vi "temperaturePanelView.vi"() -> ()   [LabVIEW 2014]
uses:
  <vilib>/LabVIEW Interface for Arduino/Type Defs/Board Type.ctl
  <vilib>/LabVIEW Interface for Arduino/Type Defs/Connection Type.ctl
  <vilib>/LabVIEW Interface for Arduino/Type Defs/Pin Mode.ctl
  <vilib>/LabVIEW Interface for Arduino/LabVIEW Interface for Arduino.lvlib
  Arduino/libraries/LIFA-DHT/DHT11.lvlib
panel:
  out "Estado del Ventilador2":bool
  out "Estado del Ventilador1":bool
  in  "Tipos de Velocidad Motor2":i8(knob) scale=0.0..3.0
  in  "Motor 2 PIN":dbl
  in  "Tipos de Velocidad Motor1":i8(knob) scale=0.0..3.0
  in  "Temperatura Considerada calor":i8
  in  "Motor 1 PIN":dbl
  out "Registro de temperatura":u8(graph)
  in  "DHT11 PIN":fxp<+,4,4>
  out "TF label":dbl
  out "Temperatura F":dbl(slide) scale=0.0..180.0
  out "TC label":dbl
  out "Temperatura C°":dbl(slide) scale=0.0..100.0
  in  "Delay":fxp<+,16,16>
  in  "stop":bool
  in  "VISA resource":refnum<visa-resource-name>
  # "Ventilador Inteligente"
  # "Arduino"
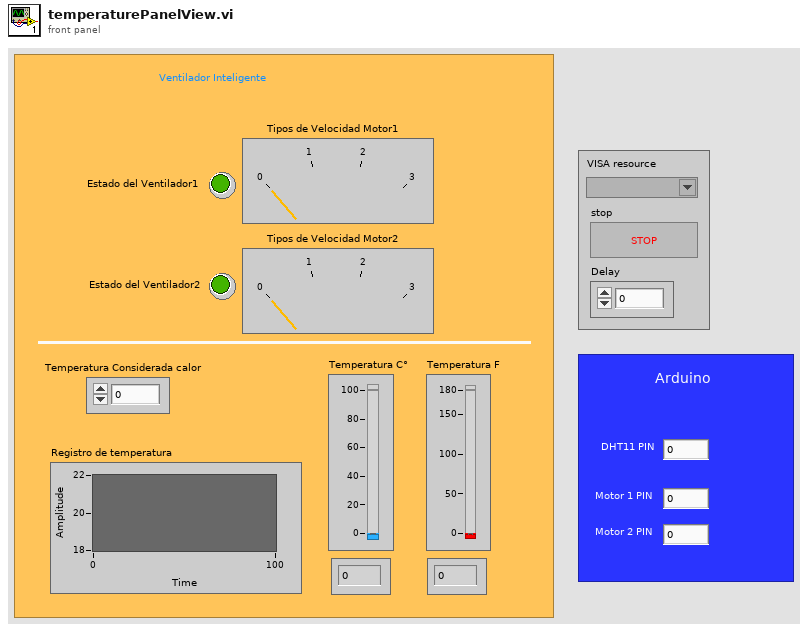
[diagram p1: front panel]
types:
  T1 = typedef "LabVIEW Interface for Arduino.lvlib/Pin Mode.ctl" = enum8{"Input", "Output"}
  T2 = typedef "LabVIEW Interface for Arduino.lvlib/Connection Type.ctl" = enum8{"USB / Serial", "XBEE", "BlueSmirf (Bluetooth)"}
  T3 = typedef "LabVIEW Interface for Arduino.lvlib/Board Type.ctl" = enum16{"Uno", "Dimuelanove w/Atmega 328", "Mega 2560"}
  T4 = typedef "LabVIEW Interface for Arduino.lvlib/Arduino Resource.ctl" = cluster{"VISA resource":refnum<visa-resource-name>, "Board Type":T3, "Connection Type":enum8{"USB / Serial"}, "Bytes Per Packet (15)":u8}
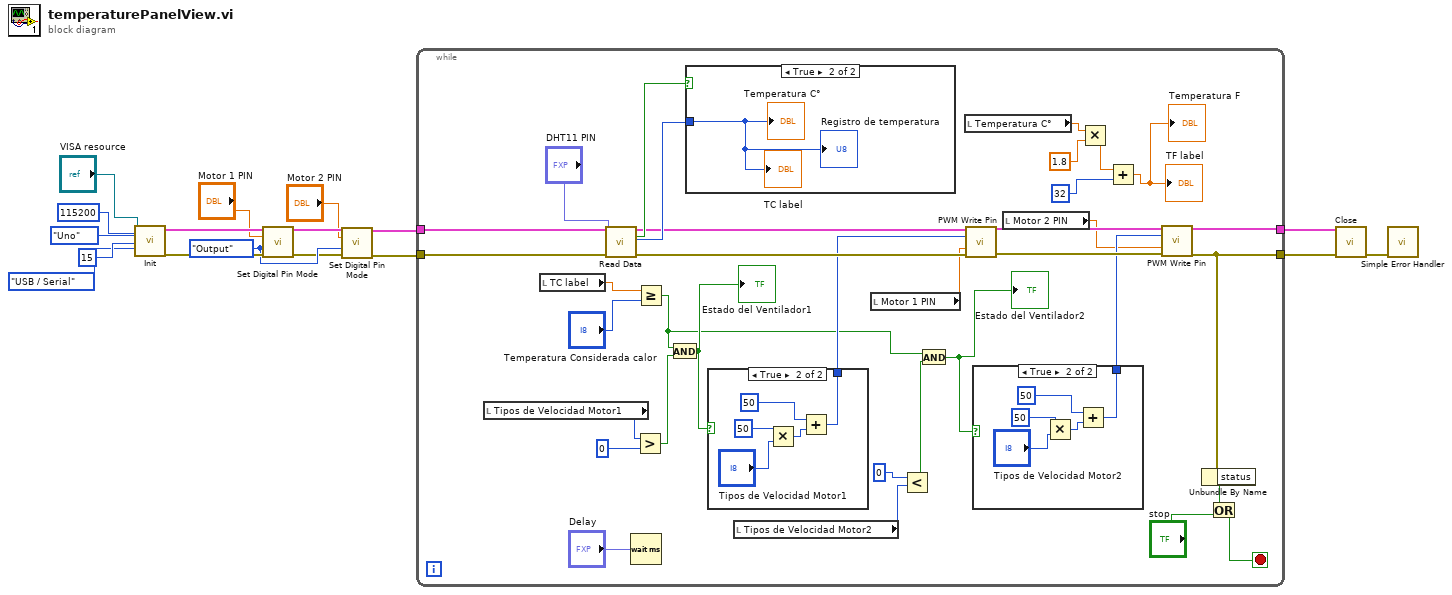
[diagram p0: block diagram]
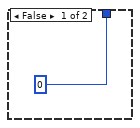
[diagram p2: hidden frame]
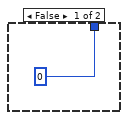
[diagram p3: hidden frame]
diagram:
  w4 = Pin_Mode."Output" ("Pin Mode (Input)")
  n1 = call <vilib>:"Init.vi"("VISA resource"="VISA resource", "Baud Rate (115200)"=u32 115200, "Board Type (Uno)"=Board_Type."Uno", "Bytes Per Packet (15)"=u32 15, "Connection Type (USB/Serial)"=Connection_Type."USB / Serial") -> ("Arduino Resource"=w9:T4, "error out"=w8:errorcluster)  [unwired: 13 in]
  n2 = call <vilib>:"Set Digital Pin Mode.vi"("Arduino Resource"=w9, "Digital I/O Pin"="Motor 1 PIN", "Pin Mode (Input)"=w4, "error in"=w8) -> ("Arduino Resource"=w6:T4, "error out"=w3:errorcluster)  [unwired: 10 in]
  n3 = call <vilib>:"Set Digital Pin Mode.vi"("Arduino Resource"=w6, "Digital I/O Pin"="Motor 2 PIN", "Pin Mode (Input)"=w4, "error in"=w3) -> ("Arduino Resource"=w5:T4, "error out"=w2:errorcluster)  [unwired: 10 in]
  n4 = while {
    tunnel: [w29] -> w12
    tunnel: [w28] -> w11
    tunnel: w5 -> [w48]
    tunnel: w2 -> [w47]
    stop <- w50 stop-if-true
    n5 = local read "Tipos de Velocidad Motor1"() -> (w32:i8)
    n6 = local read "TC label"() -> (w35:dbl)
    n7 = call "Read Data.vi"("Arduino Resource"=w48, "Pin"="DHT11 PIN", "error in (no error)"=w47) -> ("Arduino Resource"=w38:T4, "Successful?"=w46:bool, "Temperature (°C)"=w45:u8, "error out"=w37:errorcluster)  [unwired: 8 in, 1 out]
    n8 = Wait (ms)(milliseconds to wait="Delay") -> ()  [unwired: 1 out]
    n9 = Greater?(x=w32, y=0) -> (0:w26:bool)
    n10 = Greater Or Equal?(x=w35, y="Temperatura Considerada calor") -> (x >= y?=w24:bool)
    n11 = And(x=w24, y=w26) -> (x .and. y?=w25:bool)
    "Estado del Ventilador1" <- w25
    n12 = case shown="True" w46 {
      tunnel: w45 -> [_ w65]
      frame False {
      }
      frame True {
        "Temperatura C°" <- w65
        "TC label" <- w65
        "Registro de temperatura" <- w65
      }
    }
    n13 = case shown="True" w25 {
      tunnel: [0 w63] -> w33
      frame False {
      }
      frame True {
        n14 = Multiply(x=50, y="Tipos de Velocidad Motor1") -> (x*y=w62:i32)
        n15 = Add(x=50, y=w62) -> (x+y=w63:i32)
      }
    }
    n16 = local read "Tipos de Velocidad Motor2"() -> (w21:i8)
    n17 = local read "Motor 1 PIN"() -> (w36:dbl)
    n18 = Less?(x=0, y=w21) -> (x < y?=w23:bool)
    n19 = And(x=w24, y=w23) -> (x .and. y?=w20:bool)
    "Estado del Ventilador2" <- w20
    n20 = local read "Temperatura C°"() -> (w41:dbl)
    n21 = call <vilib>:"PWM Write Pin.vi"("Arduino Resource"=w38, "Duty Cycle (0 - 255)"=w33, "PWM Pin (3)"=w36, "error in"=w37) -> ("Arduino Resource"=w30:T4, "error out"=w27:errorcluster)  [unwired: 10 in]
    n22 = case shown="True" w20 {
      tunnel: [0 w55] -> w19
      frame False {
      }
      frame True {
        n23 = Multiply(x=50, y="Tipos de Velocidad Motor2") -> (x*y=w57:i32)
        n24 = Add(x=50, y=w57) -> (x+y=w55:i32)
      }
    }
    n25 = local read "Motor 2 PIN"() -> (w18:dbl)
    n26 = Multiply(x=w41, y=1.8) -> (x*y=w43:dbl)
    n27 = Add(x=w43, y=32) -> (x+y=→"Temperatura F" →"TF label":dbl)
    n28 = call <vilib>:"PWM Write Pin.vi"("Arduino Resource"=w30, "Duty Cycle (0 - 255)"=w19, "PWM Pin (3)"=w18, "error in"=w27) -> ("Arduino Resource"=w29:T4, "error out"=w28:errorcluster)  [unwired: 10 in]
    n29 = Unbundle By Name(w28) -> ("status"=w52:bool)
    n30 = Or(x=w52, y="stop") -> (x .or. y?=w50:bool)
  }
  n31 = call <vilib>:"Close.vi"("Arduino Resource"=w12, "error in"=w11) -> ("error out"=w10:errorcluster)  [unwired: 13 in]
  n32 = call <vilib>:"Simple Error Handler.vi"("error in (no error)"=w10) -> ()  [unwired: 4 in, 5 out]
